vi "OAT Envelope Detection (Waveform Output, 1 Channel).vi"(0 "scaled signal [EU]":waveform(dbl)={"t0"=timestamp(0 s since 1904-01-01), "dt"=0.0, "Y"=[]}, 1 "reset? (F)":bool, 9 "band specification":T1={"center frequency [Hz]"=4800.0, "span [Hz]"=2000.0}, 11 "error in (no error)":errorcluster) -> (4 "envelope signal [EU]":waveform(dbl), 15 "error out":errorcluster)   [LabVIEW 2017, in "SoundVib_FaultAnalysis.lvlib"]
doc: "Extracts the modulating signal, or envelope signal, from an amplitude-modulated signal. You can use the envelope detection technique to identify the mechanical faults that have amplitude-modulating effect on the vibration signal of a machine. Wire data to the <B>scaled signal [EU]</B> input to determine the polymorphic instance to use or manually select the instance."
uses:
  <vilib>/addons/Sound and Vibration/Order Analysis/Fault Analysis/SoundVib_FaultAnalysis.lvlib
  <vilib>/addons/_NISVFA/_Shared subVIs/Common/svc_Check for Waveform Parameter Continuity (no state).vi
  <vilib>/addons/Sound and Vibration/Order Analysis/Resample Order Tracking/SubVIs/oa_Calculate CIC Decimation Filter Coefficients.vi
  <vilib>/addons/Sound and Vibration/Order Analysis/Fault Analysis/SubVIs/sv_Compute Shift and Low Pass Filter with IC.vi
  <vilib>/addons/_NISVFA/_Shared subVIs/Common/svc_Get SV Channel Info.vi
  <vilib>/addons/Sound and Vibration/Order Analysis/Resample Order Tracking/SubVIs/OAT Frequency Shift (Mixer).vi
  <vilib>/addons/Sound and Vibration/Order Analysis/Resample Order Tracking/SubVIs/oa_Decimation with CIC and Compensation Filter.vi
  <vilib>/addons/Sound and Vibration/Order Analysis/Fault Analysis/SubVIs/oa_Demodulation Initial States (1 Channel).vi
  <vilib>/addons/Sound and Vibration/Order Analysis/Adv Resampling/OAT Single Stage Decimation with IC.vi
  <vilib>/addons/Sound and Vibration/Order Analysis/Resample Order Tracking/SubVIs/OAT CIC Decimation.vi
  <vilib>/addons/Sound and Vibration/Order Analysis/Resample Order Tracking/SubVIs/oa_Interpolate Zeros Between Samples.vi
  <vilib>/addons/Sound and Vibration/Order Analysis/Resample Order Tracking/SubVIs/oa_Calculate Delay of CIC Decimation Interpolation Filter.vi
  <vilib>/addons/Sound and Vibration/Order Analysis/Resample Order Tracking/SubVIs/oa_Create CIC Compensation Filter.vi
  <vilib>/addons/Sound and Vibration/Order Analysis/Resample Order Tracking/SubVIs/oa_Create CIC LP Truncation Filter.vi
  <vilib>/addons/_NISVFA/_Shared subVIs/Common/svc_Engineering Units to Unit Label.vi
  <vilib>/addons/_NISVFA/_Shared subVIs/Common/svc_Unit Label to Engineering Units.vi
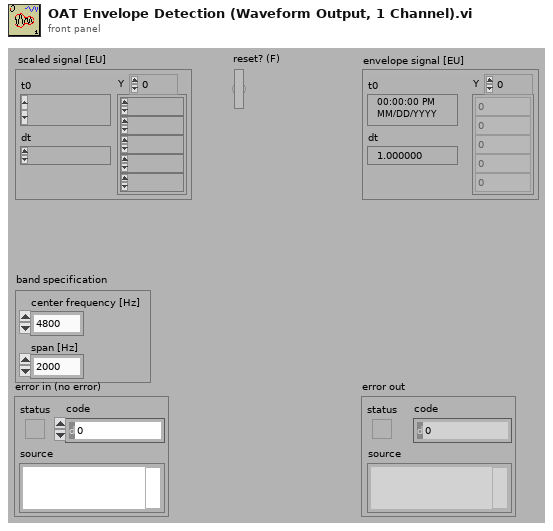
[diagram p1: front panel]
types:
  T1 = cluster{"center frequency [Hz]":dbl, "span [Hz]":dbl}
  T2 = cluster{"dt":bool, "t0 continuity":bool, "array length":bool, "channel info":bool, "name":bool}
  T3 = typedef "svc_Envelope Detection State.ctl" = cluster{"filter settings":cluster{"CIC Settings":cluster{"Numeric":i32, i32, i32}, "filters":T4[], "delay":i32, "interpolation factor":i32}, "filter state":cluster{"t0":dbl, "phase":dbl, "real filter state":cluster{cluster{dbl[]}, cluster{dbl[]}[]}, "imaginary filter state":cluster{cluster{dbl[]}, cluster{dbl[]}[]}, "delay":i32}, "reset pending":bool}
  T4 = typedef "OAT Decimation Filter.ctl" = cluster{"coefficients":dbl[], "factor":i32}
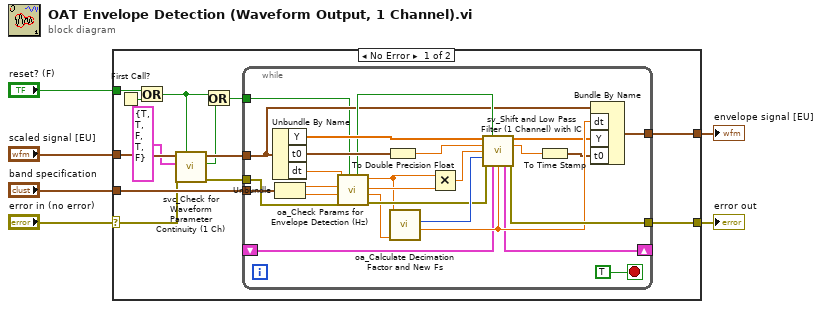
[diagram p0: block diagram]
diagram:
  n1 = case shown="No Error" "error in (no error)" {
    selector: "error in (no error)" -> [w11 w46]
    tunnel: "band specification" -> [w16 _]
    tunnel: "scaled signal [EU]" -> [w14 _]
    tunnel: [w15 w46] -> w3
    tunnel: "reset? (F)" -> [w19 _]
    tunnel: [w17 _] -> w1
    frame No Error {
      n2 = First Call?() -> (First Call?: T/F=w18:bool)
      n3 = Or(x=w19, y=w18) -> (x .or. y?=w7:bool)
      n4 = call <vilib>:"svc_Check for Waveform Parameter Continuity (1 Ch).vi"("restart averaging (F)"=w7, "error in (no error)"=w11, "checks for channel parameter change"=T2 {"dt"=TRUE, "t0 continuity"=TRUE, "array length"=FALSE, "channel info"=TRUE, "name"=FALSE}, "scaled signal [EU]"=w14) -> ("error out"=w10:errorcluster, "waveform parameter changed"=w8:bool, "dup scaled signal [EU]"=w13:waveform(dbl))  [unwired: 2 in, 3 out]
      n5 = Or(x=w7, y=w8) -> (x .or. y?=w9:bool)
      n6 = while {
        tunnel: [w45] -> w17
        tunnel: w16 -> [w44]
        tunnel: [w41] -> w15
        tunnel: w13 -> [w26]
        tunnel: w10 -> [w25]
        tunnel: w9 -> [w24]
        shift-right: [w22] -> _
        shift-left: _ -> [w21]
        stop <- TRUE stop-if-true
        n7 = Unbundle By Name(w26) -> ("Y"=w40:dbl[], "t0"=w35:timestamp, "dt"=w28:dbl)
        n8 = Unbundle(w44) -> ("center frequency [Hz]"=w32:dbl, "span [Hz]"=w31:dbl)
        n9 = call <vilib>:"oa_Check Params for Envelope Detection (Hz).vi"("reset"=w24, "error in (no error)"=w25, "span"=w31, "center"=w32, "dt"=w28) -> ("error out"=w34:errorcluster, "span out"=w30:dbl, "center out"=w29:dbl, "dt out"=w27:dbl, "reset out"=w33:bool)  [unwired: 1 in, 1 out]
        n10 = To Double Precision Float(number=w35) -> (double precision float=w38:dbl)
        n11 = call <vilib>:"oa_Calculate Decimation Factor and New Fs.vi"("span"=w30, "dt"=w27) -> ("new dt"=w39:dbl, "decimation factor"=w42:i32)  [unwired: 8 in]
        n12 = Multiply(x=w27, y=w29) -> (x*y=w43:dbl)
        n13 = call <vilib>:"sv_Shift and Low Pass Filter (1 Channel) with IC.vi"("input signal"=w40, "reset? (F)"=w33, "t0"=w38, "center"=w43, "decimation factor"=w42, "error in (no error)"=w34, "initial conditions"=w21, "new dt"=w39) -> ("enveloped signal"=w20:dbl[], "t0 out"=w37:dbl, "final conditions"=w22:T3, "error out"=w41:errorcluster)  [unwired: 4 in]
        n14 = To Time Stamp(1:w37) -> (0:w36:timestamp)
        n15 = Bundle By Name(cluster=w26, "dt"=w39, "Y"=w20, "t0"=w36) -> (w45:waveform(dbl))
      }
    }
    frame Error {
    }
  }
  "error out" <- w3
  "envelope signal [EU]" <- w1
